vi "Report_Type.vi"(8 "error in (no error)":errorcluster, 11 "IB_RestfulWS in":refnum<class "IB_RestfulWS.lvclass">) -> (0 "error out":errorcluster, 2 "type":string, 3 "IB_RestfulWS out":refnum<class "IB_RestfulWS.lvclass">)   [LabVIEW 2020, in "IB_RestfulWS.lvclass"]
uses:
  <vilib>/AppBuilder/IB_Classes/Source/Container/Build/RestfulWS/IB_RestfulWS.lvclass
  <vilib>/AppBuilder/IB_Classes/Source/Container/Build/RestfulWS/IB_RestfulWS.lvclass/IB_RestfulWS.ctl
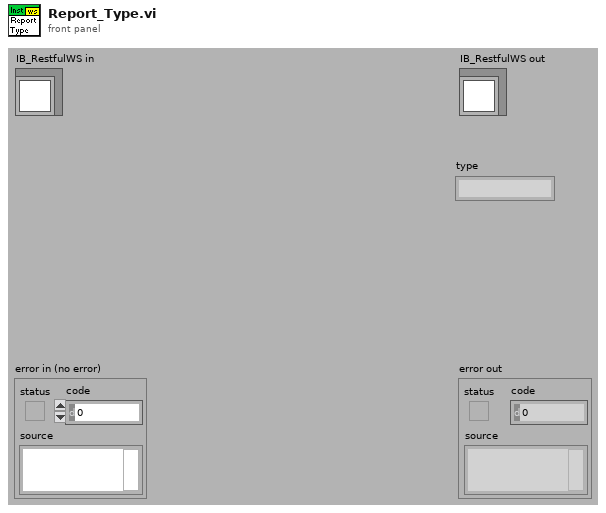
[diagram p1: front panel]
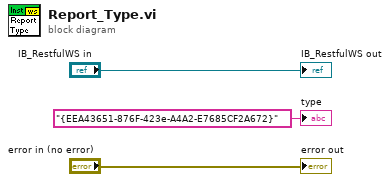
[diagram p0: block diagram]
diagram:
  "error out" <- "error in (no error)"
  "IB_RestfulWS out" <- "IB_RestfulWS in"
  "type" <- "{EEA43651-876F-423e-A4A2-E7685CF2A672}" ("type")
